vi "RollbackTransaction.vi"(8 "error in (no error)":errorcluster, 11 "SqlMapper in":refnum<class "SqlMapper.lvclass">) -> (0 "error out":errorcluster, 3 "SqlMapper out":refnum<class "SqlMapper.lvclass">)   [LabVIEW 2020, in "ORM.lvlib" / "SqlMapper.lvclass"]
uses:
  SqlMapper.lvclass
  SqlMapper.lvclass/SqlMapper.ctl
  DbConnection/DbConnection.lvclass
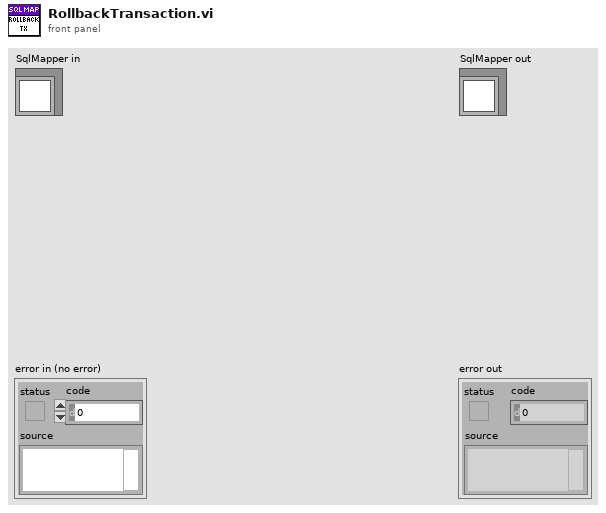
[diagram p1: front panel]
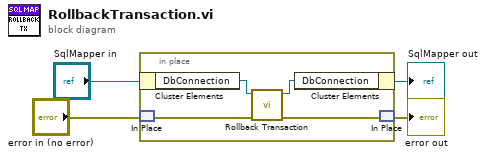
[diagram p0: block diagram]
diagram:
  n1 = in-place {
    n2 = in-place-cluster #1("SqlMapper in") -> ("DbConnection"=w8:refnum<class "DbConnection.lvclass">)
    n3 = in-place-match #2("error in (no error)") -> (w5:errorcluster)
    n4 = call "Rollback Transaction.vi"("error in (no error)"=w5, "DbConnection in"=w8) -> ("error out"=w6:errorcluster, "DbConnection out"=w7:refnum<class "DbConnection.lvclass">)  [unwired: 8 in]
    n5 = in-place-cluster #1("DbConnection"=w7) -> (→"SqlMapper out":refnum<class "SqlMapper.lvclass">)
    n6 = in-place-match #2(w6) -> (→"error out":errorcluster)
  }
